vi "NEW Ping stock FPGA.vi"() -> ()   [LabVIEW 2018]
uses:
  <vilib>/myRIO/Instrument Drivers/Onboard IO/DIO/typedefs/DIO Reference.ctl
  <vilib>/myRIO/Common/Instrument Driver Framework/Utilities/typedefs/myRIO Generic Hardware Reference.ctl
  <vilib>/myRIO/Common/Instrument Driver Framework/Utilities/typedefs/Hardware Version Enum.ctl
  <vilib>/myRIO/Common/Instrument Driver Framework/Utilities/typedefs/myRIO v1.0 Reference.ctl
  <vilib>/myRIO/Common/Instrument Driver Framework/Utilities/typedefs/Generic FPGA Reference.ctl
  <vilib>/myRIO/Common/Instrument Driver Framework/myRIO v1.0/DIO/typedefs/DIO Channels List.ctl
  <vilib>/myRIO/Common/Instrument Driver Framework/myRIO v1.0/DIO/typedefs/DIO Channels Enum.ctl
  <vilib>/userdefined/High Color/nirio_resource_hc.ctl
  <vilib>/myRIO/Common/Instrument Driver Framework/myRIO v1.0/DIO/vis/myRIO v1.1 Open DIO.vi
  <vilib>/myRIO/Common/Instrument Driver Framework/Utilities/vis/Validate Channels.vi
  <vilib>/myRIO/Common/Instrument Driver Framework/myRIO v1.0/DIO/vis/myRIO v1.0 Reserve DIO.vi
  <vilib>/myRIO/Common/Instrument Driver Framework/myRIO v1.0/DIO/vis/myRIO v1.0 Close DIO.vi
  <vilib>/myRIO/Common/Instrument Driver Framework/myRIO v1.0/Resource Manager/vis/myRIO v1.0 Reserve Channel List.vi
  <vilib>/myRIO/Common/Instrument Driver Framework/myRIO v1.0/DIO/vis/myRIO v1.0 Build MUX Configuration DIO.vi
  <vilib>/myRIO/Common/Instrument Driver Framework/myRIO v1.0/DIO/vis/myRIO v1.0 Unreserve DIO.vi
  <vilib>/myRIO/Common/Instrument Driver Framework/myRIO v1.0/Resource Manager/vis/myRIO v1.0 Reserve Channel.vi
  <vilib>/myRIO/Common/Instrument Driver Framework/myRIO v1.0/Resource Manager/vis/myRIO v1.0 Unreserve Channel.vi
  <vilib>/myRIO/Common/Instrument Driver Framework/myRIO v1.0/Resource Manager/vis/myRIO v1.0 Create Configuration List.vi
  <vilib>/myRIO/Common/Instrument Driver Framework/myRIO v1.0/Resource Manager/vis/myRIO v1.0 Unreserve Channel List.vi
  <vilib>/myRIO/Common/Instrument Driver Framework/myRIO v1.0/Resource Manager/vis/myRIO v1.0 Build Mutex Name.vi
  <vilib>/Utility/VariantDataType/GetNumericInfo.vi
  <vilib>/Utility/error.llb/Error Cluster From Error Code.vi
  <vilib>/myRIO/Common/Instrument Driver Framework/myRIO v1.0/myRIO v1.1 Open.vi
  <vilib>/myRIO/Common/Instrument Driver Framework/Utilities/vis/IO Manager.vi
  <vilib>/myRIO/Common/Instrument Driver Framework/Utilities/vis/Configuration Manager.vi
  <vilib>/myRIO/Common/Instrument Driver Framework/myRIO v1.0/Resource Manager/vis/myRIO v1.0 Configure IO.vi
  <vilib>/myRIO/Common/Instrument Driver Framework/myRIO v1.0/myRIO v1.0 Close.vi
  <vilib>/myRIO/Common/Instrument Driver Framework/myRIO v1.0/DIO/vis/myRIO v1.0 Write DIO.vi
  <vilib>/myRIO/Common/Instrument Driver Framework/myRIO v1.0/DIO/vis/myRIO v1.0 Read DIO.vi
  <vilib>/myRIO/Common/Instrument Driver Framework/myRIO v1.0/DIO/vis/myRIO v1.0 Shutdown DIO.vi
  <vilib>/myRIO/Instrument Drivers/Onboard IO/DIO/vis/myRIO DIO Open.xnode
  <vilib>/myRIO/Instrument Drivers/Onboard IO/DIO/DIO.lvlib
panel:
  out "Waveform Chart":dbl(graph)
  out "error out":errorcluster
  in  "stop":bool
  out "Tick Count(uSec)":u32
  out "Distance":dbl
  out "Enum":T1(ring)
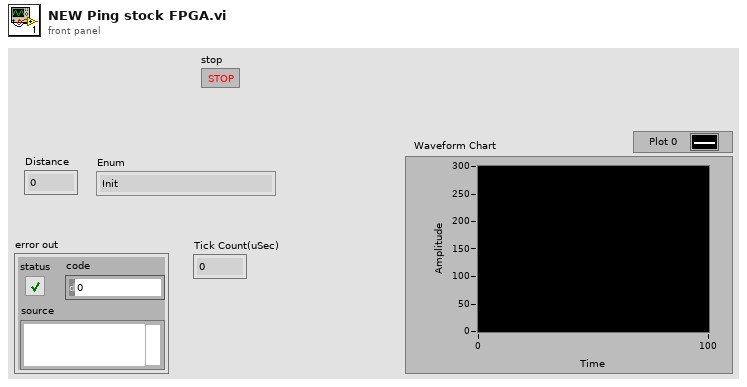
[diagram p1: front panel]
types:
  T1 = enum16{"Init", "Input Trigger Pulse", "Echo Holdoff", "Wait for pulse", "Delay before next"}
  T2 = typedef "DIO.lvlib/DIO Reference.ctl" = cluster{"myRIO Reference":T3, "DIO Channels List":T7}
  T3 = typedef "myRIO Generic Hardware Reference.ctl" = cluster{"myRIO Model":T4, "myRIO Hardware Reference":T5}
  T4 = typedef "Hardware Version Enum.ctl" = enum16{"Unknown", "myRIO-1900", "myRIO-1950", "roboRIO", "NI ELVIS RIO CM", "ELVIS III"}
  T5 = typedef "myRIO v1.0 Reference.ctl" = cluster{"Generic FPGA Reference":T6, "Allow multiple opens":bool}
  T6 = typedef "Generic FPGA Reference.ctl" = refnum<k20>
  T7 = typedef "DIO Channels List.ctl" = T8[]
  T8 = typedef "DIO Channels Enum.ctl" = enum16{"Not Connected", "C/DIO0", "C/DIO1", "C/DIO2", "C/DIO3", "C/DIO4", "C/DIO5", "C/DIO6", "C/DIO7", "A/DIO0", "A/DIO1", "A/DIO2", "A/DIO3", "A/DIO4", "A/DIO5", "A/DIO6", "A/DIO7", "A/DIO8", "A/DIO9", "A/DIO10", "A/DIO11", "A/DIO12", "A/DIO13", "A/DIO14", "A/DIO15", "A/DIO16", "A/DIO17", "A/DIO18", "A/DIO19", "B/DIO0", "B/DIO1", "B/DIO2", "B/DIO3", "B/DIO4", "B/DIO5", "B/DIO6", "B/DIO7", "B/DIO8", "B/DIO9", "B/DIO10", "B/DIO11", "B/DIO12", "B/DIO13", "B/DIO14", "B/DIO15", "B/DIO16", "B/DIO17", "B/DIO18", "B/DIO19", "LED0", "LED1", "LED2", "LED3", "Button0", "DIO/DIO0", "DIO/DIO1", "DIO/DIO2", "DIO/DIO3", "DIO/DIO4", "DIO/DIO5", "DIO/DIO6", "DIO/DIO7", "DIO/DIO8", "DIO/DIO9", "SPI/CS0", "SPI/CS1", "SPI/CS2", "SPI/CS3", "LED RADIO (Green)", "LED RADIO (Red)", "LED COMM (Green)", "LED COMM (Red)", "LED MODE (Green)", "LED MODE (Red)"}
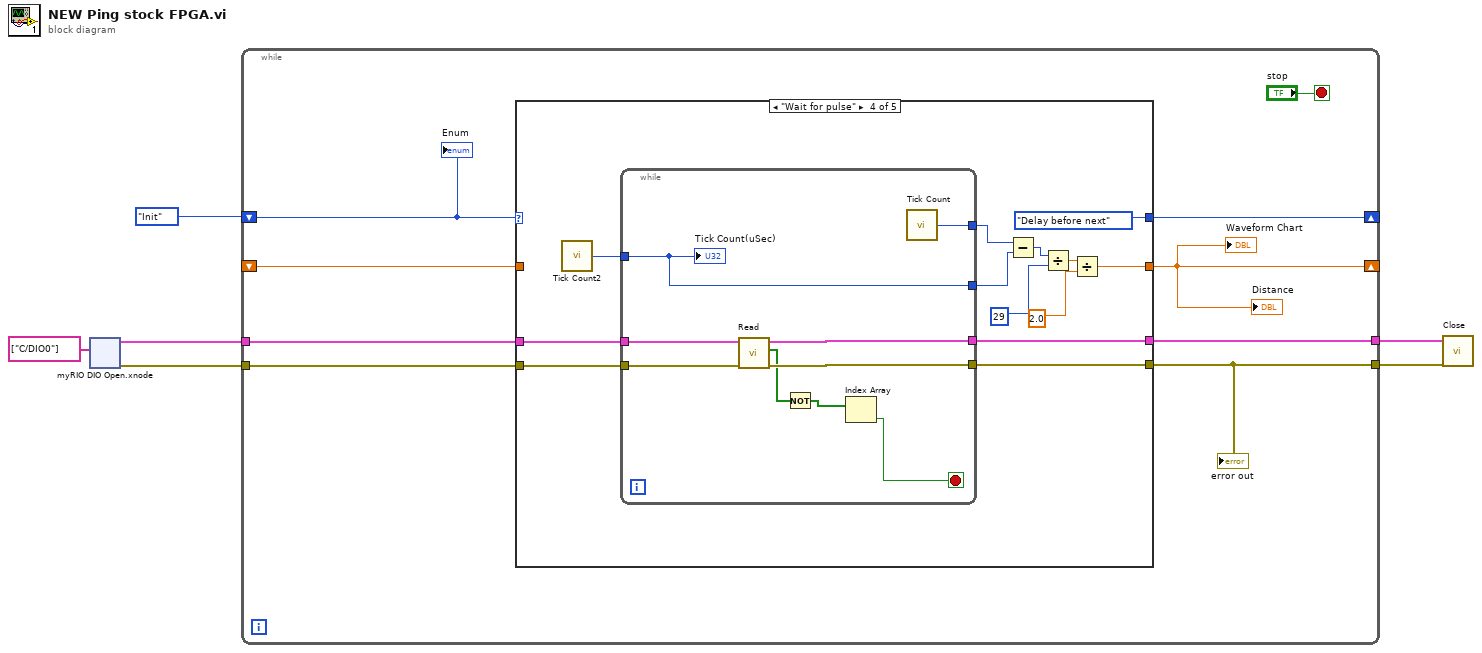
[diagram p0: block diagram]
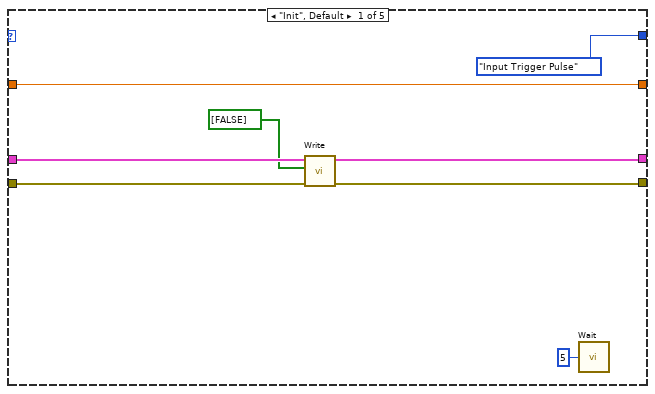
[diagram p2: hidden frame]
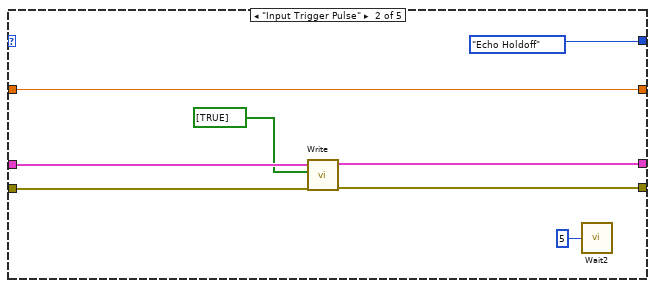
[diagram p3: hidden frame]
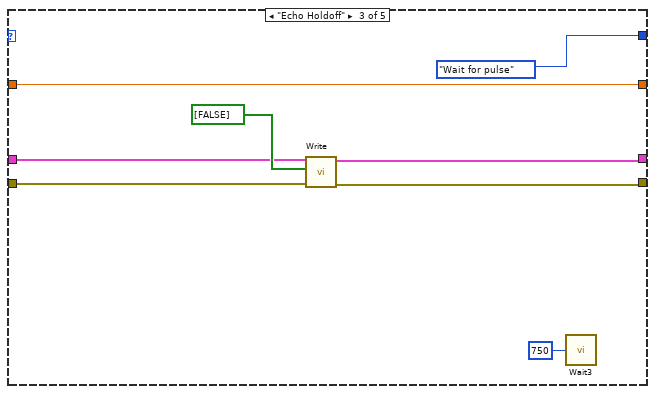
[diagram p4: hidden frame]
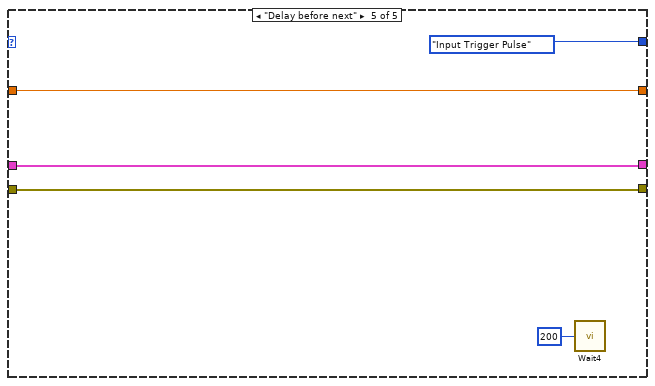
[diagram p5: hidden frame]
diagram:
  n1 = xnode "myRIO DIO Open.xnode"("Channel Names"=tag[] ["C/DIO0"]) -> ("error out"=w4:errorcluster, "DIO Ref Out"=w3:T2)  [unwired: 2 in]
  n2 = while {
    shift-right: [w13] -> _
    shift-left: T1."Init" -> [w14]
    shift-right: [w7] -> _
    shift-left: _ -> [w12]
    tunnel: w4 -> [w10]
    tunnel: w3 -> [w11]
    tunnel: [w9] -> w2
    tunnel: [w8] -> w1
    stop <- "stop" stop-if-true
    n3 = case shown="\"Wait for pulse\"" w14 {
      tunnel: [T1."Input Trigger Pulse" T1."Echo Holdoff" T1."Wait for pulse" T1."Delay before next" T1."Input Trigger Pulse"] -> w13
      tunnel: [w21 w29 w37 w45 w66] -> w7
      tunnel: w12 -> [w21 w29 w37 _ w66]
      tunnel: w11 -> [w19 w28 w35 w43 w63]
      tunnel: w10 -> [w20 w27 w34 w41 w62]
      tunnel: [w17 w26 w32 w42 w63] -> w9
      tunnel: [w16 w25 w33 w40 w62] -> w8
      frame "Init", Default {
        n4 = call <vilib>:"Write.vi"("error in (no error)"=w20, "Values"=bool[] [FALSE], "DIO Ref In"=w19) -> ("error out"=w16:errorcluster, "DIO Ref Out"=w17:T2)  [unwired: 6 in]
        n5 = call "Wait"("Count(uSec)"=u32 5) -> ()  [unwired: 1 out]
      }
      frame "Input Trigger Pulse" {
        n6 = call <vilib>:"Write.vi"("error in (no error)"=w27, "Values"=bool[] [TRUE], "DIO Ref In"=w28) -> ("error out"=w25:errorcluster, "DIO Ref Out"=w26:T2)  [unwired: 6 in]
        n7 = call "Wait2"("Count(uSec)"=u32 5) -> ()  [unwired: 1 out]
      }
      frame "Echo Holdoff" {
        n8 = call <vilib>:"Write.vi"("error in (no error)"=w34, "Values"=bool[] [FALSE], "DIO Ref In"=w35) -> ("error out"=w33:errorcluster, "DIO Ref Out"=w32:T2)  [unwired: 6 in]
        n9 = call "Wait3"("Count(uSec)"=u32 750) -> ()  [unwired: 1 out]
      }
      frame "Wait for pulse" {
        n10 = call "Tick Count2"() -> ("Tick Count(uSec)"=w52:u32)
        n11 = while {
          tunnel: w52 -> [w60]
          tunnel: [w61] -> w51
          tunnel: [w60] -> w50
          tunnel: w43 -> [w59]
          tunnel: [w58] -> w42
          tunnel: w41 -> [w57]
          tunnel: [w56] -> w40
          stop <- w53 stop-if-true
          n12 = call <vilib>:"Read.vi"("error in (no error)"=w57, "DIO Ref In"=w59) -> ("error out"=w56:errorcluster, "Values"=w55:bool[], "DIO Ref Out"=w58:T2)  [unwired: 7 in]
          n13 = Not(x=w55) -> (.not. x?=w54:bool[])
          n14 = Index Array(array=w54) -> (element=w53:bool)  [unwired: 1 in]
          n15 = call "Tick Count"() -> ("Tick Count(uSec)"=w61:u32)
          "Tick Count(uSec)" <- w60
        }
        n16 = Subtract(x=w51, y=w50) -> (x-y=w49:u32)
        n17 = Divide(x=w49, y=u32 29) -> (x/y=w47:dbl)
        n18 = Divide(x=w47, y=2.0) -> (x/y=w45:dbl)
      }
      frame "Delay before next" {
        n19 = call "Wait4"("Count(uSec)"=u32 200) -> ()  [unwired: 1 out]
      }
    }
    "Distance" <- w7
    "error out" <- w8
    "Waveform Chart" <- w7
    "Enum" <- w14
  }
  n20 = call <vilib>:"Close.vi"("error in (no error)"=w1, "DIO Ref In"=w2) -> ()  [unwired: 9 in, 1 out]
